vi "Elevator Notify Autonomous.vi"(8 "error in (no error)":errorcluster, 9 "Notify when settled?":bool, 10 "Settled?":bool, 11 "State":T1) -> (0 "error out":errorcluster)   [LabVIEW 2014]
uses:
  Elevator States.ctl
  Robot Global Data.vi
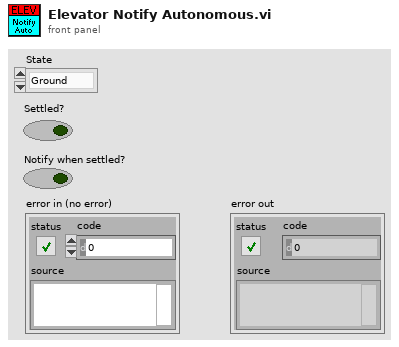
[diagram p1: front panel]
types:
  T1 = typedef "Elevator States.ctl" = enum16{"Ground", "Tote 1", "Tote 2", "Tote 3", "Tote 4", "Tote 5", "Tote 6"}
  T2 = typedef "WPI_DriverStationRobotMode2.ctl" = enum16{"Autonomous Disabled", "Autonomous Enabled", "Teleop Disabled", "Teleop Enabled", "Disconnected", "Finish", "Test Disabled", "Test Enabled", "Emergency Stopped"}
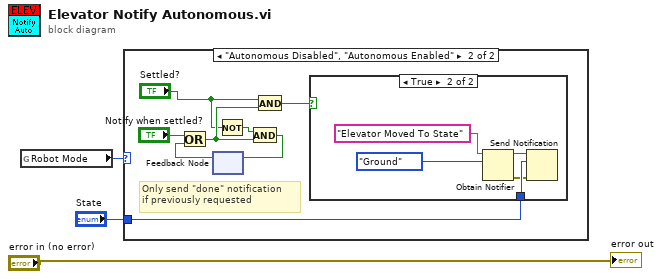
[diagram p0: block diagram]
diagram:
  n1 = global read "Robot Global Data.vi" "Robot Mode"() -> (w3:T2)
  n2 = case shown="\"Autonomous Disabled\", \"Autonomous Enabled\"" w3 {
    tunnel: "State" -> [_ w7]
    frame Default {
    }
    frame "Autonomous Disabled", "Autonomous Enabled" {
      # "Only send \"done\" notification\nif previously requested"
      n3 = feedback #1() -> (w8:bool)  [unwired: 1 in]
      n4 = Or(x="Notify when settled?", y=w8) -> (x .or. y?=w6:bool)
      n5 = Not(x="Settled?") -> (.not. x?=w10:bool)
      n6 = And(x=w10, y=w6) -> (x .and. y?=w9:bool)
      n7 = feedback-in #1(w9) -> ()
      n8 = And(x="Settled?", y=w6) -> (x .and. y?=w5:bool)
      n9 = case shown="True" w5 {
        tunnel: w7 -> [_ w14]
        frame False {
        }
        frame True {
          n10 = Obtain Notifier(name (unnamed)="Elevator Moved To State", notification data type=Elevator_States."Ground" ("Output State")) -> (notifier out=w15:refnum<notifier>, error out=w13:errorcluster)  [unwired: 2 in, 1 out]
          n11 = Send Notification(notification=w14, notifier=w15, error in (no error)=w13) -> ()  [unwired: 2 out]
        }
      }
    }
  }
  "error out" <- "error in (no error)"
